vi "Reset.vi"() -> (3 "Boolean":bool)   [LabVIEW 2014]
uses:
  Support Files/Global Data!!!.vi
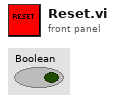
[diagram p1: front panel]
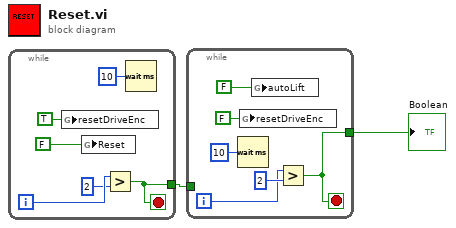
[diagram p0: block diagram]
diagram:
  n1 = while {
    tunnel: [w5] -> w1
    i -> [w7]
    stop <- w5 stop-if-true
    n2 = global write "Global Data!!!.vi" "resetDriveEnc"(TRUE ("resetDriveEnc")) -> ()
    n3 = global write "Global Data!!!.vi" "Reset"(FALSE ("resetDriveEnc")) -> ()
    n4 = Greater?(x=w7, y=2) -> (0:w5:bool)
    n5 = Wait (ms)(milliseconds to wait=u32 10) -> ()  [unwired: 1 out]
  }
  n6 = while {
    tunnel: w1 -> [_]
    tunnel: [w11] -> w2
    i -> [w12]
    stop <- w11 stop-if-true
    n7 = Wait (ms)(milliseconds to wait=u32 10) -> ()  [unwired: 1 out]
    n8 = global write "Global Data!!!.vi" "resetDriveEnc"(FALSE ("resetDriveEnc")) -> ()
    n9 = global write "Global Data!!!.vi" "autoLift"(FALSE ("resetDriveEnc")) -> ()
    n10 = Greater?(x=w12, y=2) -> (0:w11:bool)
  }
  "Boolean" <- w2
